vi "Varian Magnet (No Objects).vi"(8 "error in (no error)":errorcluster) -> (0 "error out":errorcluster, 3 "Varian Magnet out":T1={"Fluke VISA resource name"="GPIB0::2::INSTR", "DAQ Physical Channel"="Dev1/ao0", "DAQ Task - Set"="", "DAQ Task - Read"="", "Control Voltage"=enum."40V", "extrapolated"={"x locations"=[], "coefficients"=[]}, "last 5 field numbers"=[], "Fluke Multimeter"={"function (0:volts DC)"=0, "range (0:auto)"=0, "rate (0:slow)"=0, "trigger mode (0:internal)"=0, "Autorange"=FALSE}} {"Fluke Multimeter"."function (0:volts DC)" items=["volts DC", "volts AC", "2-wire k.ohms", "4-wire k.ohms", "mA DC", "mA AC"]; "Fluke Multimeter"."range (0:auto)" items=["autorange", "200mV, 200 ohms", "2V, 2 kohms", "20V, 20 kohms", "200V, 200 kohms", "1000Vdc, 700 Vac, 2 Mohms", "20 Mohms"]; "Fluke Multimeter"."rate (0:slow)" items=["slow", "medium", "fast"]; "Fluke Multimeter"."trigger mode (0:internal)" items=["internal - continuous trigger", "external - rear panel trigger with delay", "external - bus trigger with delay", "external - rear panel trigger", "external - bus trigger"]})   [LabVIEW 2012]
uses:
  Global/GPIB Numbers.vi
  <vilib>/DAQmx/create/channels.llb/DAQmx Create Channel (AO-Voltage-Basic).vi
  <vilib>/DAQmx/create/channels.llb/DAQmx Create Channel (AI-Voltage-Basic).vi
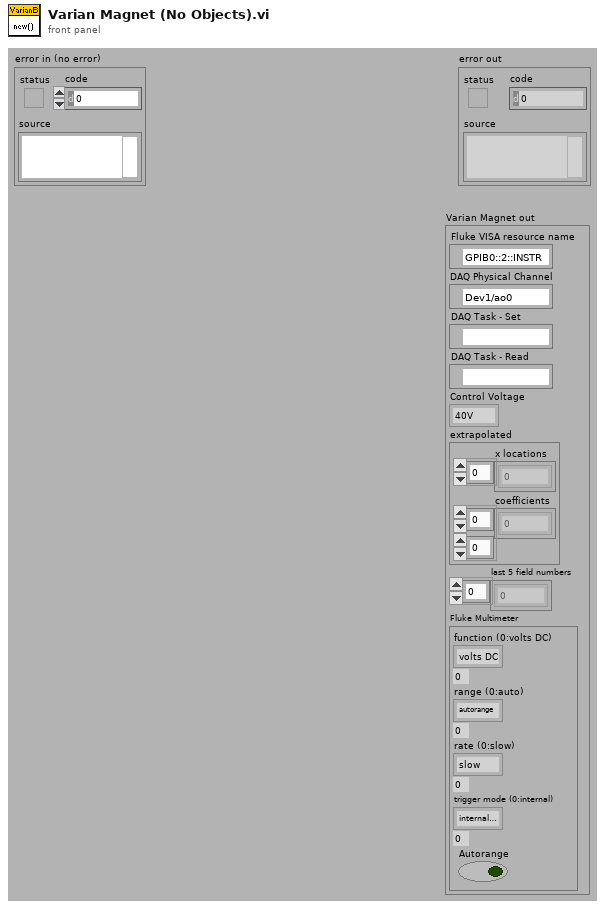
[diagram p1: front panel]
types:
  T1 = cluster{"Fluke VISA resource name":refnum<visa-resource-name>, "DAQ Physical Channel":tag, "DAQ Task - Set":refnum<k21>, "DAQ Task - Read":refnum<k21>, "Control Voltage":enum16{"Please Select a Value", "30V", "40V"}, "extrapolated":cluster{"x locations":dbl[], "coefficients":dbl[][]}, "last 5 field numbers":dbl[], "Fluke Multimeter":cluster{"function (0:volts DC)":u16, "range (0:auto)":u16, "rate (0:slow)":u16, "trigger mode (0:internal)":u16, "Autorange":bool}}
  T2 = cluster{"function (0:volts DC)":u16, "range (0:auto)":u16, "rate (0:slow)":u16, "trigger mode (0:internal)":u16, "Autorange":bool}
  T3 = cluster{"function (0:volts DC)":i16, "range (0:auto)":i16, "rate (0:slow)":i16, "trigger mode (0:internal":i16, "Autorange":bool}
  T4 = typedef "GPIB Type Def.ctl" = cluster{"Name":string, "bus":dbl, "GPIB":dbl, "GPIB as string":string, "byte":i32, "VISA Resource Name":refnum<visa-resource-name>}
  T5 = typedef "NI_Gmath.lvlib/in_piecewise interp poly control.ctl" = cluster{"x locations":dbl[], "coefficients":dbl[][]}
  T6 = cluster{"Fluke VISA resource name":refnum<visa-resource-name>, "DAQ Physical Channel":tag, "DAQ Task - Set":refnum<k21>, "DAQ Task - Read":refnum<k21>, "Control Voltage":enum16{"Please Select a Value", "30V", "40V"}, "extrapolated":T5, "last 5 field numbers":dbl[], "Fluke Multimeter":cluster{"function (0:volts DC)":u16, "range (0:auto)":u16, "rate (0:slow)":u16, "trigger mode (0:internal)":u16, "Autorange":bool}}
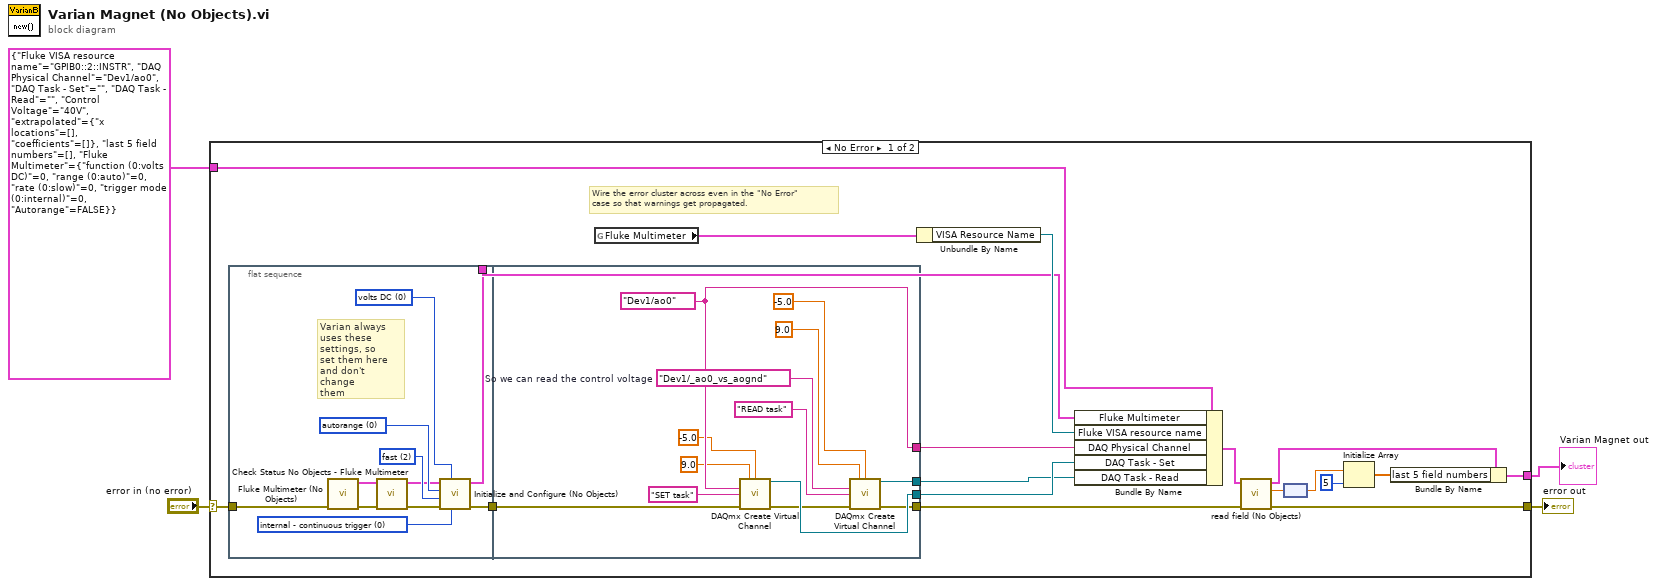
[diagram p0: block diagram]
diagram:
  n1 = case shown="No Error" "error in (no error)" {
    selector: "error in (no error)" -> [w22 w48]
    tunnel: [w12 w48] -> w3
    tunnel: [w9 w47] -> w1
    tunnel: T1 {"Fluke VISA resource name"="GPIB0::2::INSTR", "DAQ Physical Channel"="Dev1/ao0", "DAQ Task - Set"="", "DAQ Task - Read"="", "Control Voltage"=enum."40V", "extrapolated"={"x locations"=[], "coefficients"=[]}, "last 5 field numbers"=[], "Fluke Multimeter"={"function (0:volts DC)"=0, "range (0:auto)"=0, "rate (0:slow)"=0, "trigger mode (0:internal)"=0, "Autorange"=FALSE}} ("Varian Magnet in") -> [w21 w47]
    frame No Error {
      # "Wire the error cluster across even in the \"No Error\"\ncase so that warnings get propagated."
      n2 = flat-sequence {
        tunnel: w22 -> [w33]
        tunnel: [w30] -> w18
        tunnel: [w25] -> w17
        tunnel: w18 -> [w46]
        tunnel: [w40] -> w13
        tunnel: [w45] -> w15
        tunnel: [w44] -> w16
        tunnel: [w41] -> w14
        frame #0 {
          w26 = u16 0 items=["volts DC", "volts AC", "2-wire k.ohms", "4-wire k.ohms", "mA DC", "mA AC"] ("function (0:volts DC)")
          w27 = u16 0 items=["autorange", "200mV, 200 ohms", "2V, 2 kohms", "20V, 20 kohms", "200V, 200 kohms", "1000Vdc, 700 Vac, 2 Mohms", "20 Mohms", "20 mV, 20 ohms"] ("range (0:auto)")
          w28 = u16 2 items=["slow", "medium", "fast"] ("rate (0:slow)")
          w29 = u16 0 items=["internal - continuous trigger", "external - rear panel trigger with delay", "external - bus trigger with delay", "external - rear panel trigger", "external - bus trigger"] ("trigger mode (0:internal)")
          # "Varian always\nuses these\nsettings, so\nset them here\nand don't change\nthem"
          n3 = call "Fluke Multimeter (No Objects).vi"("error in (no error)"=w33) -> ("error out"=w32:errorcluster, "Fluke Multimeter out"=w24:T2)  [unwired: 9 in]
          n4 = call "Check Status No Objects - Fluke Multimeter.vi"("error in (no error)"=w32, "input cluster"=w24) -> ("error out"=w31:errorcluster, "output cluster"=w23:T3)  [unwired: 6 in, 2 out]
          n5 = call "Initialize and Configure (No Objects).vi"("trigger mode (0:internal)"=w29, "function (0:volts DC)"=w26, "error in (no error)"=w31, "rate (0:slow)"=w28, "range (0:auto)"=w27, "input cluster"=w23) -> ("error out"=w30:errorcluster, "output cluster"=w25:T3)  [unwired: 4 in]
        }
        frame #1 {
          w43 = tag "Dev1/_ao0_vs_aognd"  # So we can read the control voltage
          w44 = tag "Dev1/ao0" ("physical channels")
          n6 = call-poly <vilib>:"DAQmx Create Virtual Channel.vi"("maximum value"=9.0, "minimum value"=-5.0, "physical channels"=w44, "name to assign"="SET task", "error in"=w46) -> ("task out"=w45:refnum<k21>, "error out"=w42:errorcluster)  [unwired: 4 in, 5 out]
          n7 = call-poly <vilib>:"DAQmx Create Virtual Channel.vi"("maximum value"=9.0, "minimum value"=-5.0, "physical channels"=w43, "name to assign"="READ task", "error in"=w42) -> ("task out"=w41:refnum<k21>, "error out"=w40:errorcluster)  [unwired: 4 in, 5 out]
        }
      }
      n8 = global read "GPIB Numbers.vi" "Fluke Multimeter"() -> (w20:T4)
      n9 = Unbundle By Name(w20) -> ("VISA Resource Name"=w19:refnum<visa-resource-name>)
      n10 = Bundle By Name(cluster=w21, "Fluke Multimeter"=w17, "Fluke VISA resource name"=w19, "DAQ Physical Channel"=w16, "DAQ Task - Set"=w15, "DAQ Task - Read"=w14) -> (w5:T1)
      n11 = call "read field (No Objects).vi"("error in (no error)"=w13, "Varian Magnet In"=w5) -> ("error out"=w12:errorcluster, "Field"=w7:dbl[unit], "Varian Magnet Out"=w10:T6)  [unwired: 7 in]
      n12 = node(w7) -> (w6:dbl)
      n13 = Initialize Array(w6, 5 ("dimension size")) -> (w8:dbl[])
      n14 = Bundle By Name(cluster=w10, "last 5 field numbers"=w8) -> (w9:T6)
    }
    frame Error {
    }
  }
  "error out" <- w3
  "Varian Magnet out" <- w1
